vi "Start_PE7265.vi"(0 "Lock-in Reference":u16, 1 "VI-Pfad":path) -> ()   [LabVIEW 2019]
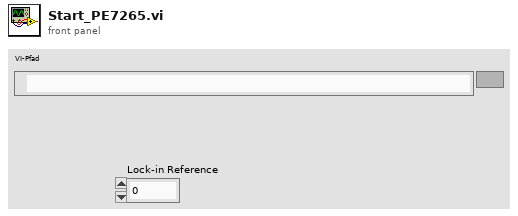
[diagram p1: front panel]
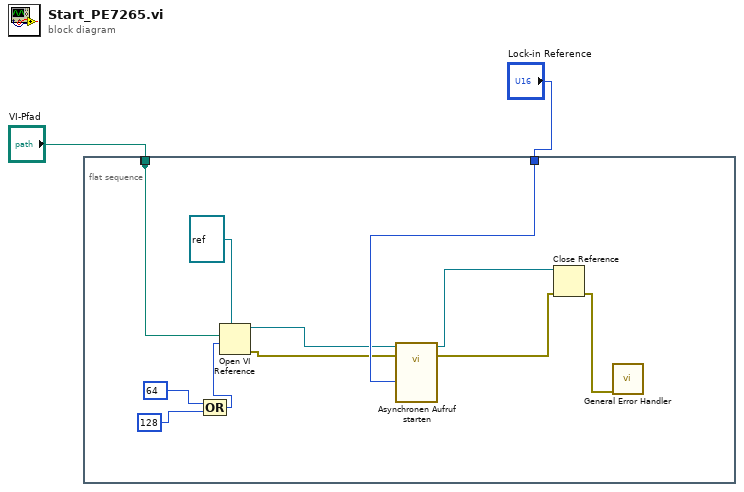
[diagram p0: block diagram]
diagram:
  n1 = flat-sequence {
    tunnel: [w4] -> _
    tunnel: "VI-Pfad" -> [w4]
    tunnel: "Lock-in Reference" -> [w13]
    frame #0 {
      n2 = Compound Arithmetic op=OR(64 ("options"), 128 ("options")) -> (w3:i32)
      n3 = Open VI Reference(type specifier VI Refnum (for type only)=refnum<vi> refnum, vi path=w4, options=w3) -> (vi reference=w11:refnum<vi>, error out=w12:errorcluster)  [unwired: 3 in]
      n4 = call-by-ref "Asynchronen Aufruf starten"(reference=w11, error in=w12, "Lock-in Reference"=w13) -> (reference out=w10:refnum<vi>, error out=w9:errorcluster)
      n5 = Close Reference(reference=w10, error in (no error)=w9) -> (error out=w8:errorcluster)
      n6 = call <vilib>:"General Error Handler.vi"("error in (no error)"=w8) -> ()  [unwired: 10 in, 5 out]
    }
  }
